vi "Drive SS Outputs 2016.vi"(10 "Drive Actuator Values In":T1) -> (0 "error out":errorcluster)   [LabVIEW 2015]
uses:
  Drive Actuator Values Out.ctl
  <vilib>/Rock Robotics/WPI/CAN/TalonSRX/WPI_CANTalonSRX_APIControlMode.ctl
  <vilib>/Rock Robotics/WPI/Solenoid/WPI_SolenoidValue.ctl
  Global Variables/refnum names.vi
  <vilib>/Rock Robotics/WPI/Solenoid/WPI_SolenoidSetEnum.vi
  Global Variables/Temp Variables.vi
panel:
  out "appended array":dbl[](array[numeric])
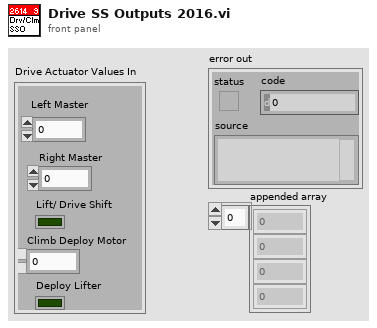
[diagram p1: front panel]
types:
  T1 = typedef "Drive Actuator Values Out.ctl" = cluster{"Left Master":dbl, "Right Master":dbl, "Lift/ Drive Shift":bool, "Climb Deploy Motor":dbl, "Deploy Lifter":bool}
  T2 = typedef "WPI_SolenoidValue.ctl" = enum16{"Off", "On", "Forward", "Reverse"}
  T3 = typedef "WPI_CANTalonSRX_APIControlMode.ctl" = enum8{"Percent VBus", "Speed", "Position", "Slave", "Unchanged / Invalid", "Voltage Compensation", "Current", "Motion Profile"}
  T4 = typedef "WPI_MotorControlDeviceRef.ctl" = cluster{"DeviceStatus":errorcluster, "Type":T5, "PWM":cluster{"PWM Channel":T6, "DeadBand":T7}, "CAN":cluster{"Device Number":u8, "Control Mode":T8, "Semaphore":T9, "Max Vout":dbl, "TalonSRX Control Mode":T3}, "Invert":bool}
  T5 = typedef "WPI_MotorControlType.ctl" = enum16{"PWM", "CAN", "CANTalonSRX"}
  T6 = typedef "FPGA_DIOPWMChannel.ctl" = enum8{"PWM 0", "PWM 1", "PWM 2", "PWM 3", "PWM 4", "PWM 5", "PWM 6", "PWM 7", "PWM 8", "PWM 9", "PWM MXP 0", "PWM MXP 1", "PWM MXP 2", "PWM MXP 3", "PWM MXP 4", "PWM MXP 5", "PWM MXP 6", "PWM MXP 7", "PWM MXP 8", "PWM MXP 9", "Invalid"}
  T7 = typedef "WPI_PWMDeadband.ctl" = cluster{"Name":string, "maxPositivePwm":i32, "minPositivePwm":i32, "centerPwm":i32, "maxNegativePwm":i32, "minNegativePwm":i32, "angularRange":u16}
  T8 = typedef "WPI_CANJaguar_ControlMode.ctl" = enum8{"Percent VBus", "Current", "Speed", "Position", "Voltage"}
  T9 = typedef "Semaphore RefNum" = refnum<k1>
  T10 = typedef "WPI_SolenoidDevRef.ctl" = cluster{"DevStatus":errorcluster, "Pneumatics Control Module":u8, "Forward Solenoid Channel":T11, "Reverse Solenoid Channel":T11}
  T11 = typedef "WPI_SolenoidChannel.ctl" = enum8{"Solenoid 0", "Solenoid 1", "Solenoid 2", "Solenoid 3", "Solenoid 4", "Solenoid 5", "Solenoid 6", "Solenoid 7", "Invalid"}
  T12 = typedef "WPI_CANTalonSRX_GlobalStatus.ctl" = cluster{"Applied Throttle":dbl, "Module Enabled":bool, "CAN Error":errorcluster, "Closed Loop Error":dbl, "Forward Limit Switch Closed":bool, "Reverse Limit Switch Closed":bool, "Sensor Position":dbl, "Sensor Velocity":dbl, "Current":dbl, "Sticky Fault - Over Temp":bool, "Sticky Fault - Under Voltage":bool, "Sticky Fault - Forward Limit":bool, "Sticky Fault - Reverse Limit":bool, "Sticky Fault - Forward Soft Limit":bool, "Sticky Fault - Reverse Soft Limit":bool, "Brake is Enabled":bool, "Encoder Position":dbl, "Encoder Velocity":dbl, "Encoder Index Count":dbl, "Encoder A Pin State":bool, "Encoder B Pin State":bool, "Encoder Index Pin State":bool, "Analog In":dbl, "Analog In Velocity":dbl, "Temperature (C)":dbl, "Battery Voltage":dbl, "Control 5 Is Supported":bool, "Current Profile Slot Select":dbl, "Pos Div 8":bool, "Vel Div 4":bool, "Pulse Width Position":i32, "Pulse Width Velocity":i32, "Pulse Width Rise To Rise (us)":i32, "Pulse Width Rise To Fall (us)":i32, "Mot Prof Active Is Under Run":bool, "Mot Prof Active Has Under Run":bool, "Mot Prof Active Is Last":bool, "Mot Prof Active Velocity Only":bool, "Mot Prof Active Is Valid":bool, "Mot Prof Buffer Is Full":bool, "Mot Prof Active Profile Slot Select":i32, "Mot Prof NextID":i32, "Mot Prof Count":i32, "Mot Prof Active Velocity":dbl, "Mot Prof Active Position":dbl, "Mot Prof Output Enable":i32}
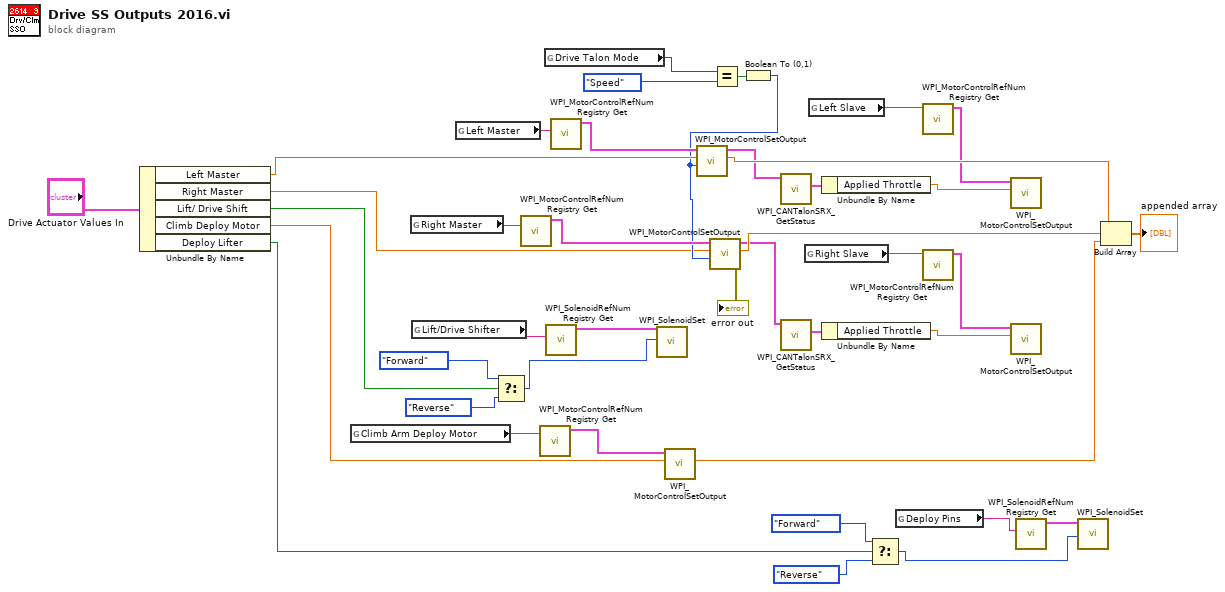
[diagram p0: block diagram]
diagram:
  n1 = Unbundle By Name("Drive Actuator Values In") -> ("Left Master"=w37:dbl, "Right Master"=w3:dbl, "Lift/ Drive Shift"=w29:bool, "Climb Deploy Motor"=w34:dbl, "Deploy Lifter"=w2:bool)
  n2 = global read "refnum names.vi" "Climb Arm Deploy Motor"() -> (w36:string)
  n3 = global read "refnum names.vi" "Right Master"() -> (w39:string)
  n4 = global read "refnum names.vi" "Lift/Drive Shifter"() -> (w33:string)
  n5 = global read "refnum names.vi" "Left Master"() -> (w40:string)
  n6 = Select(t=WPI_SolenoidValue."Forward" ("Value"), s=w29, f=WPI_SolenoidValue."Reverse" ("Value")) -> (s? t:f=w28:T2)
  n7 = call <vilib>:"WPI_MotorControlRefNum Registry Get.vi"("refnum name"=w39) -> ("MotorControlDevRef"=w38:T4)  [unwired: 9 in, 1 out]
  n8 = call <vilib>:"WPI_MotorControlRefNum Registry Get.vi"("refnum name"=w36) -> ("MotorControlDevRef"=w35:T4)  [unwired: 9 in, 1 out]
  n9 = global read "Temp Variables.vi" "Drive Talon Mode"() -> (w23:T3)
  n10 = call <vilib>:"WPI_SolenoidRefNum Registry Get.vi"("refnum name"=w33) -> ("SolenoidDevRef"=w32:T10)  [unwired: 9 in, 1 out]
  n11 = call <vilib>:"WPI_MotorControlRefNum Registry Get.vi"("refnum name"=w40) -> ("MotorControlDevRef"=w27:T4)  [unwired: 9 in, 1 out]
  n12 = call-poly <vilib>:"WPI_SolenoidSet.vi"("Value"=w28, "SolenoidDevRef"=w32) -> ()  [unwired: 8 in, 2 out]
  n13 = call <vilib>:"WPI_MotorControlSetOutput.vi"("Output"=w34, "MotorControlDevRef"=w35) -> ("Motor Output"=w1:dbl)  [unwired: 7 in, 2 out]
  n14 = Equal?(x=w23, y=WPI_CANTalonSRX_APIControlMode."Speed" ("Drive Talon Mode")) -> (x = y?=w26:bool)
  n15 = Boolean To (0,1)(Boolean=w26) -> (0, 1=w25:i16)
  n16 = call <vilib>:"WPI_MotorControlSetOutput.vi"("Sync Group / Parameter Slot"=w25, "Output"=w37, "MotorControlDevRef"=w27) -> ("Motor Output"=w21:dbl, "MotorControlDevRef"=w17:T4)  [unwired: 6 in, 1 out]
  n17 = call <vilib>:"WPI_MotorControlSetOutput.vi"("Sync Group / Parameter Slot"=w25, "Output"=w3, "MotorControlDevRef"=w38) -> ("error out"=→"error out":errorcluster, "Motor Output"=w20:dbl, "MotorControlDevRef"=w9:T4)  [unwired: 6 in]
  n18 = call <vilib>:"WPI_CANTalonSRX_GetStatus.vi"("CAN Talon SRX Ref"=w17) -> ("Talon SRX Status"=w16:T12)  [unwired: 8 in, 2 out]
  n19 = call <vilib>:"WPI_CANTalonSRX_GetStatus.vi"("CAN Talon SRX Ref"=w9) -> ("Talon SRX Status"=w11:T12)  [unwired: 8 in, 2 out]
  n20 = global read "refnum names.vi" "Right Slave"() -> (w10:string)
  n21 = global read "refnum names.vi" "Left Slave"() -> (w18:string)
  n22 = Unbundle By Name(w16) -> ("Applied Throttle"=w14:dbl)
  n23 = Unbundle By Name(w11) -> ("Applied Throttle"=w13:dbl)
  n24 = Select(t=WPI_SolenoidValue."Forward" ("Value"), s=w2, f=WPI_SolenoidValue."Reverse" ("Value")) -> (s? t:f=w4:T2)
  n25 = global read "refnum names.vi" "Deploy Pins"() -> (w5:string)
  n26 = call <vilib>:"WPI_MotorControlRefNum Registry Get.vi"("refnum name"=w18) -> ("MotorControlDevRef"=w15:T4)  [unwired: 9 in, 1 out]
  n27 = call <vilib>:"WPI_MotorControlRefNum Registry Get.vi"("refnum name"=w10) -> ("MotorControlDevRef"=w12:T4)  [unwired: 9 in, 1 out]
  n28 = call <vilib>:"WPI_MotorControlSetOutput.vi"("Output"=w14, "MotorControlDevRef"=w15) -> ()  [unwired: 7 in, 3 out]
  n29 = call <vilib>:"WPI_MotorControlSetOutput.vi"("Output"=w13, "MotorControlDevRef"=w12) -> ()  [unwired: 7 in, 3 out]
  n30 = call <vilib>:"WPI_SolenoidRefNum Registry Get.vi"("refnum name"=w5) -> ("SolenoidDevRef"=w6:T10)  [unwired: 9 in, 1 out]
  n31 = call-poly <vilib>:"WPI_SolenoidSet.vi"("Value"=w4, "SolenoidDevRef"=w6) -> ()  [unwired: 8 in, 2 out]
  n32 = Build Array(w21, w20, w1) -> (→"appended array":dbl[])
